vi "Configure Basic Digital Generator.vi"(0 "VISA resource name":refnum<visa-resource-name>, 1 "Enable AB Lock (T: Enable)":bool=TRUE, 2 "Gain (100 %)":dbl=100.0, 3 "Invert (T: Enable)":bool=TRUE, 5 "Channel (0: A)":i32(ring) items=["A", "B"], 7 "Output Mode (0: Stereo)":i32(ring) items=["Stereo", "Mono"], 9 "Dither (0: dgNoDither)":i32(ring) items=["dgNoDither", "dgTriangular", "dgRectangular"], 11 "error in (no error)":errorcluster, 12 "Auto On (T: Enable)":bool=TRUE, 13 "Enable Waveform (T: Enable)":bool=TRUE) -> (4 "VISA resource name out":refnum<visa-resource-name>, 15 "error out":errorcluster)   [LabVIEW 2014, in "Stanford Research SR1.lvlib"]
doc: "Configures the basic attributes of the Digital Audio Generator."
uses:
  Stanford Research SR1.lvlib
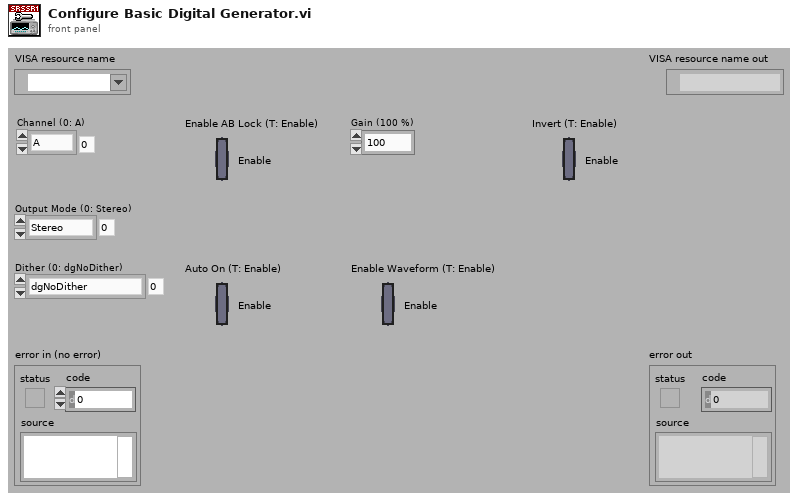
[diagram p1: front panel]
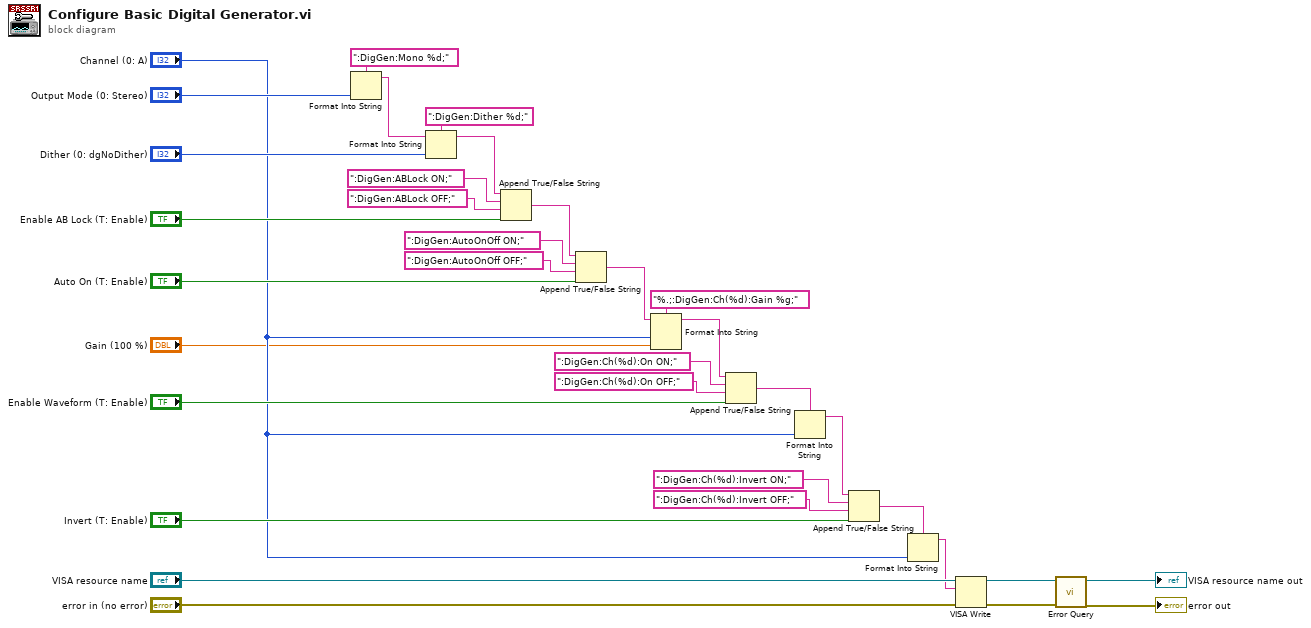
[diagram p0: block diagram]
diagram:
  n1 = Format Into String(format string=":DigGen:Mono %d;", "Output Mode (0: Stereo)") -> (resulting string=w32:string)  [unwired: 2 in, 1 out]
  n2 = Format Into String(format string=":DigGen:Dither %d;", initial string=w32, "Dither (0: dgNoDither)") -> (resulting string=w29:string)  [unwired: 1 in, 1 out]
  n3 = Append True/False String(1:"Enable AB Lock (T: Enable)", 2:":DigGen:ABLock OFF;", 3:":DigGen:ABLock ON;", 4:w29) -> (0:w25:string)
  n4 = Append True/False String(1:"Auto On (T: Enable)", 2:":DigGen:AutoOnOff OFF;", 3:":DigGen:AutoOnOff ON;", 4:w25) -> (0:w21:string)
  n5 = Format Into String(format string="%.;:DigGen:Ch(%d):Gain %g;", initial string=w21, "Channel (0: A)", "Gain (100 %)") -> (resulting string=w19:string)  [unwired: 1 in, 1 out]
  n6 = Append True/False String(1:"Enable Waveform (T: Enable)", 2:":DigGen:Ch(%d):On OFF;", 3:":DigGen:Ch(%d):On ON;", 4:w19) -> (0:w6:string)
  n7 = Format Into String(format string=w6, "Channel (0: A)") -> (resulting string=w5:string)  [unwired: 2 in, 1 out]
  n8 = Append True/False String(1:"Invert (T: Enable)", 2:":DigGen:Ch(%d):Invert OFF;", 3:":DigGen:Ch(%d):Invert ON;", 4:w5) -> (0:w4:string)
  n9 = Format Into String(format string=w4, "Channel (0: A)") -> (resulting string=w3:string)  [unwired: 2 in, 1 out]
  n10 = VISA Write(VISA resource name="VISA resource name", write buffer=w3, error in (no error)="error in (no error)") -> (VISA resource name out=w10:refnum<visa-resource-name>, error out=w9:errorcluster)  [unwired: 1 out]
  n11 = call "Error Query.vi"("error in (no error)"=w9, "VISA resource name"=w10) -> ("error out"=→"error out":errorcluster, "VISA resource name out"=→"VISA resource name out":refnum<visa-resource-name>)  [unwired: 6 in, 2 out]
